vi "Single Unbounded.vi"() -> ()   [LabVIEW 2022 SP3]
uses:
  Flex/Publish Element.vi
  Flex/Instantiate.vi
  Flex/))Channel.vi
  Flex/Check Room in Queues.vi
  Flex/Flex.lvlib
panel:
  in  "Second Lossless":bool
  out "Count 2":i32
  out "Chart 2":i32(graph)
  in  "With Lossy":bool
  in  "With Event":bool
  out "Queued Count":i32[](array[numeric])
  out "Chart":i32(graph)
  out "Count":i32
  in  "stop":bool
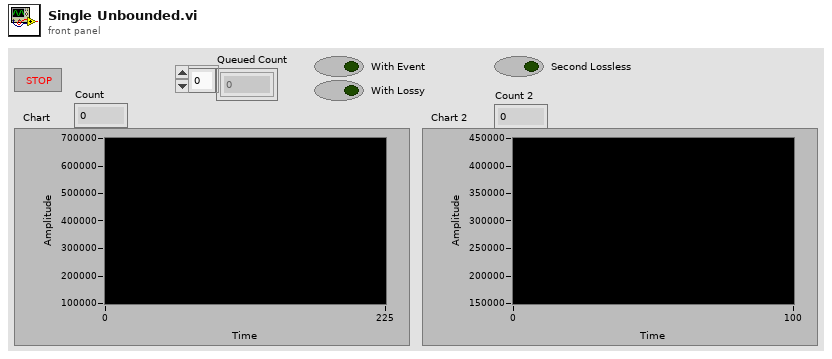
[diagram p1: front panel]
types:
  T1 = typedef "Flex.lvlib/))Channel.ctl" = refnum<queue>
  T2 = typedef "Flex.lvlib/Element.ctl" = dbl
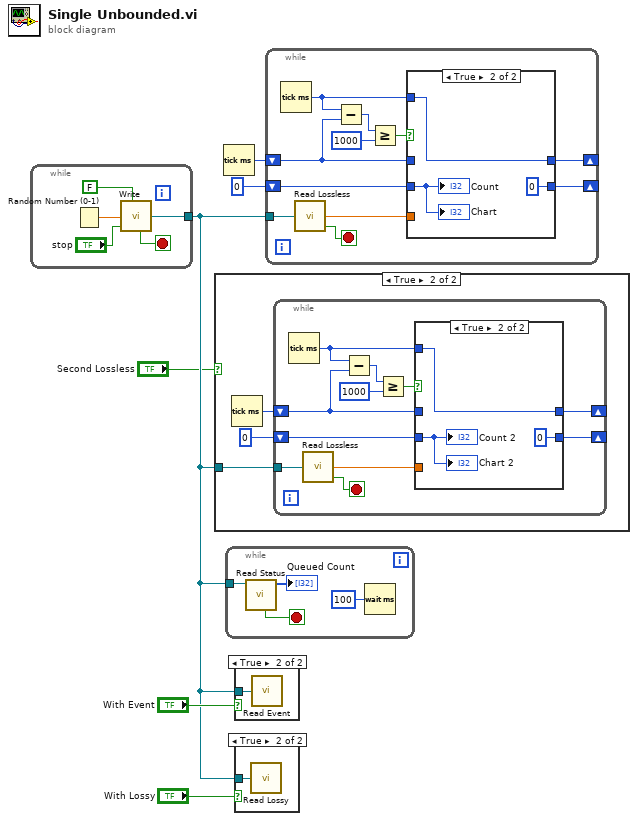
[diagram p0: block diagram]
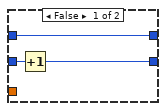
[diagram p3: hidden frame]
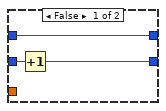
[diagram p4: hidden frame]
diagram:
  n1 = while {
    tunnel: [w8] -> w2
    stop <- w9 stop-if-true
    n2 = Random Number (0-1)() -> (number: 0 to 1=w11:dbl)
    n3 = call "Write.vi"("Synchronous (F)"=FALSE, "element"=w11, "Close? (F)"="stop") -> ("channel"=w8:T1, "Closed?"=w9:bool)  [unwired: 4 in, 1 out]
  }
  n4 = case shown="True" "Second Lossless" {
    tunnel: w2 -> [_ w12]
    frame False {
    }
    frame True {
      n5 = Tick Count (ms)() -> (millisecond timer value=w14:u32)
      n6 = while {
        tunnel: w12 -> [w25]
        shift-right: [w16] -> _
        shift-left: w14 -> [w20]
        shift-right: [w17] -> _
        shift-left: 0 -> [w18]
        stop <- w24 stop-if-true
        n7 = Tick Count (ms)() -> (millisecond timer value=w15:u32)
        n8 = call "Read Lossless.vi"("FlexChannel"=w25) -> ("Element"=w19:T2, "Closed?"=w24:bool)  [unwired: 6 in, 1 out]
        n9 = Subtract(x=w15, y=w20) -> (x-y=w23:u32)
        n10 = Greater Or Equal?(x=w23, y=u32 1000) -> (x >= y?=w21:bool)
        n11 = case shown="True" w21 {
          tunnel: w20 -> [w26 _]
          tunnel: w19 -> [_ _]
          tunnel: w18 -> [w28 w29]
          tunnel: [w27 0] -> w17
          tunnel: [w26 w31] -> w16
          tunnel: w15 -> [_ w31]
          frame False {
            n12 = Increment(x=w28) -> (x+1=w27:i32)
          }
          frame True {
            "Count 2" <- w29
            "Chart 2" <- w29
          }
        }
      }
    }
  }
  n13 = Tick Count (ms)() -> (millisecond timer value=w6:u32)
  n14 = while {
    tunnel: w2 -> [w35]
    stop <- w33 stop-if-true
    n15 = call "Read Status.vi"("channel"=w35) -> ("Queued Count"=→"Queued Count":i32[], "Closed?"=w33:bool)  [unwired: 2 in, 7 out]
    n16 = Wait (ms)(milliseconds to wait=u32 100) -> ()  [unwired: 1 out]
  }
  n17 = case shown="True" "With Event" {
    tunnel: w2 -> [_ w36]
    frame False {
    }
    frame True {
      n18 = call "Read Event.vi"("FlexChannel"=w36) -> ()  [unwired: 8 in, 1 out]
    }
  }
  n19 = case shown="True" "With Lossy" {
    tunnel: w2 -> [_ w37]
    frame False {
    }
    frame True {
      n20 = call "Read Lossy.vi"("FlexChannel"=w37) -> ()  [unwired: 4 in, 5 out]
    }
  }
  n21 = while {
    tunnel: w2 -> [w48]
    shift-right: [w39] -> _
    shift-left: w6 -> [w43]
    shift-right: [w40] -> _
    shift-left: 0 -> [w41]
    stop <- w47 stop-if-true
    n22 = Tick Count (ms)() -> (millisecond timer value=w38:u32)
    n23 = call "Read Lossless.vi"("FlexChannel"=w48) -> ("Element"=w42:T2, "Closed?"=w47:bool)  [unwired: 6 in, 1 out]
    n24 = Subtract(x=w38, y=w43) -> (x-y=w46:u32)
    n25 = Greater Or Equal?(x=w46, y=u32 1000) -> (x >= y?=w44:bool)
    n26 = case shown="True" w44 {
      tunnel: w43 -> [w49 _]
      tunnel: w42 -> [_ _]
      tunnel: w41 -> [w51 w52]
      tunnel: [w50 0] -> w40
      tunnel: [w49 w54] -> w39
      tunnel: w38 -> [_ w54]
      frame False {
        n27 = Increment(x=w51) -> (x+1=w50:i32)
      }
      frame True {
        "Count" <- w52
        "Chart" <- w52
      }
    }
  }
